vi "HR_Zones_Calculate.vi"(8 "error in (no error)":errorcluster, 11 "wejœcie":T1={"Runer's Data"={"Name"="", "Age"=0}, "HR Max"=0, "Raw Data"={"Time"=[], "Bpm"=[]}, "% HR MAX "=[], "HR Zones "=[], "no of points"=[], "Heart Rate Zone No 2"=[1, 2, 3, 4, 5]}) -> (0 "error out":errorcluster, 2 "x*y":dbl[](array[numeric]), 3 "wyjœcie":T1={"Runer's Data"={"Name"="", "Age"=0}, "HR Max"=0, "Raw Data"={"Time"=[], "Bpm"=[]}, "% HR MAX "=[], "HR Zones "=[], "no of points"=[], "Heart Rate Zone No 2"=[1, 2, 3, 4, 5]})   [LabVIEW 2024]
uses:
  klaster 4.ctl
  klaster.ctl
  klaster 2.ctl
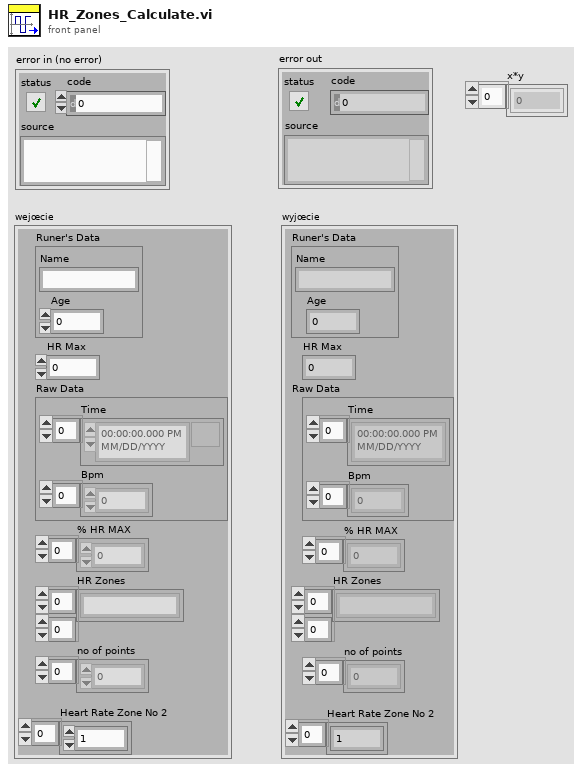
[diagram p1: front panel]
types:
  T1 = typedef "klaster 4.ctl" = cluster{"Runer's Data":T2, "HR Max":i32, "Raw Data":T3, "% HR MAX ":dbl[], "HR Zones ":string[][], "no of points":dbl[], "Heart Rate Zone No 2":i32[]}
  T2 = typedef "klaster.ctl" = cluster{"Name":string, "Age":i32}
  T3 = typedef "klaster 2.ctl" = cluster{"Time":timestamp[], "Bpm":i32[]}
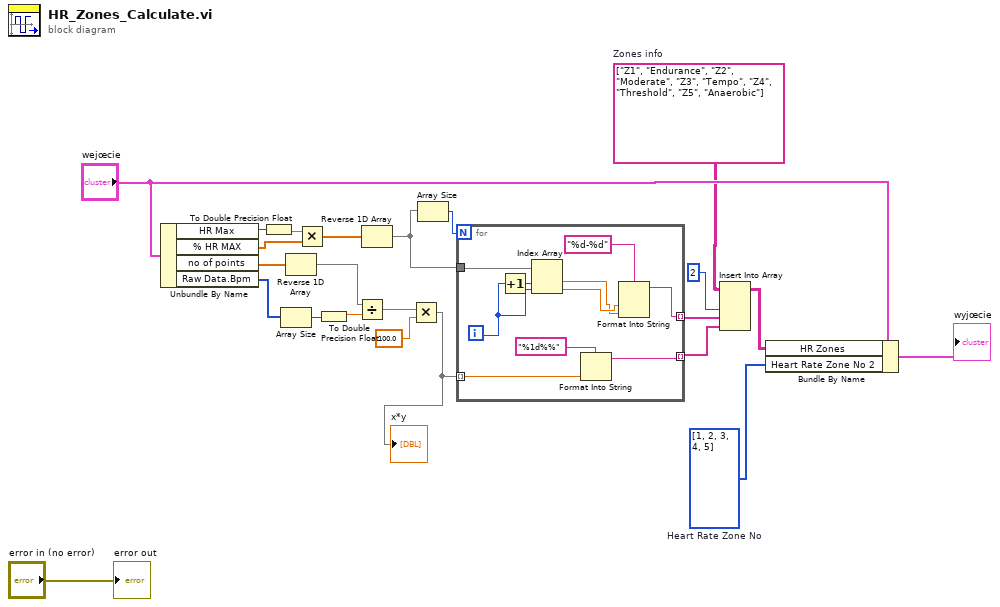
[diagram p0: block diagram]
diagram:
  w1 = string[][] [["Z1", "Endurance"], ["Z2", "Moderate"], ["Z3", "Tempo"], ["Z4", "Threshold"], ["Z5", "Anaerobic"]]  # Zones info
  w10 = i32[] [1, 2, 3, 4, 5]  # Heart Rate Zone No
  n1 = Unbundle By Name("wejœcie") -> ("HR Max"=w2:i32, "% HR MAX"=w14:dbl[], "no of points"=w13:dbl[], "Raw Data.Bpm"=w8:i32[])
  n2 = To Double Precision Float(number=w2) -> (double precision float=w3:dbl)
  n3 = Array Size(array=w8) -> (size(s)=w7:i32)
  n4 = Reverse 1D Array(array=w13) -> (reversed array=w21:dbl[])
  n5 = Multiply(x=w3, y=w14) -> (x*y=w15:dbl[])
  n6 = To Double Precision Float(number=w7) -> (double precision float=w6:dbl)
  n7 = Divide(x=w21, y=w6) -> (x/y=w16:dbl[])
  n8 = Reverse 1D Array(array=w15) -> (reversed array=w19:dbl[])
  n9 = Multiply(x=w16, y=100.0) -> (x*y=w11:dbl[])
  "x*y" <- w11
  n10 = Array Size(array=w19) -> (size(s)=w20:i32)
  n11 = for {
    N: w20 -> [_]
    tunnel: w19 -> [w33]
    tunnel: w11 -> [w29] mode=indexing
    tunnel: [w28] -> w22 mode=indexing
    tunnel: [w26] -> w23 mode=indexing
    i -> [w31]
    n12 = Increment(x=w31) -> (x+1=w32:i32)
    n13 = Index Array(array=w33, index #1=w32, index #2=w31) -> (element #1=w24:dbl, element #2=w25:dbl)
    n14 = Format Into String(format string="%1d%%", w29) -> (resulting string=w26:string)  [unwired: 2 in, 1 out]
    n15 = Format Into String(format string="%d-%d", w25, w24) -> (resulting string=w28:string)  [unwired: 2 in, 1 out]
  }
  n16 = Insert Into Array(array=w1, index (col)=2 ("disabled index (col)"), new element #1=w22, new element #2=w23) -> (w9:string[][])  [unwired: 1 in]
  n17 = Bundle By Name(cluster="wejœcie", "HR Zones"=w9, "Heart Rate Zone No 2"=w10) -> (→"wyjœcie":T1)
  "error out" <- "error in (no error)"
